vi "Set He Line Interlock Configuration.vi"(8 "error in (no error)":errorcluster, 9 "Manual Mode (False)":bool, 10 "Open? (False)":bool, 11 "He Line in":refnum<class "He Line.lvclass">) -> (0 "error out":errorcluster, 1 "Interlock Chain":refnum<class "Interlock Chain.lvclass">, 2 "Open? (False) 2":bool, 3 "He Line out":refnum<class "He Line.lvclass">)   [LabVIEW 2015, in "cRIO-Carbondioxide.lvlib" / "CO2-Actor.lvlib" / "He Line.lvclass"]
uses:
  He Line.lvclass
  Interlocks/Interlock Chain/Interlock Chain.lvclass
  cRIO-CO2/cRIO-CO2.lvclass
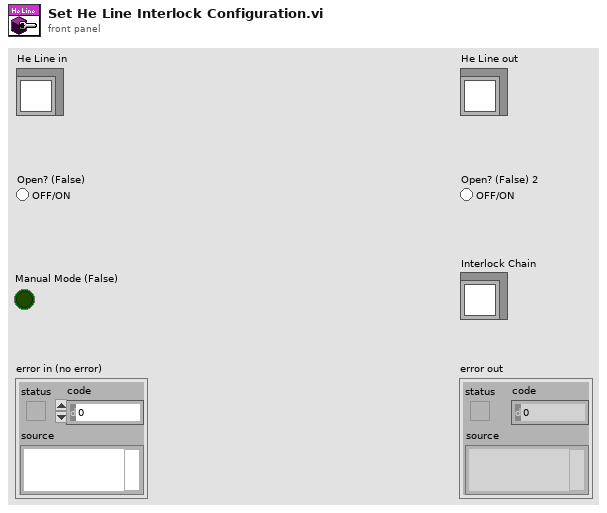
[diagram p1: front panel]
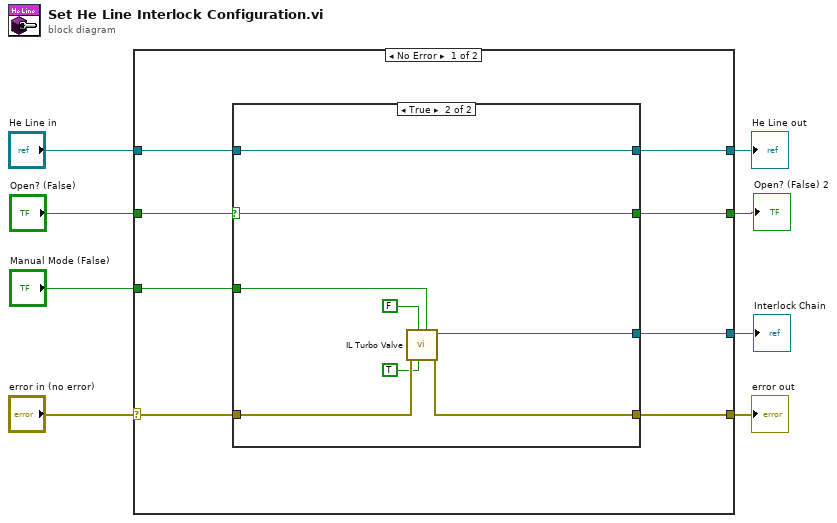
[diagram p0: block diagram]
diagram:
  n1 = case shown="No Error" "error in (no error)" {
    selector: "error in (no error)" -> [w16 w29]
    tunnel: [w15 w29] -> w7
    tunnel: [w11 w28] -> w5
    tunnel: "He Line in" -> [w12 w28]
    tunnel: "Open? (False)" -> [w10 _]
    tunnel: [w14 _] -> w3
    tunnel: "Manual Mode (False)" -> [w13 _]
    tunnel: [w9 _] -> w1
    frame No Error {
      n2 = case shown="True" w10 {
        selector: w10 -> [w17 w21]
        tunnel: w16 -> [w19 w27]
        tunnel: [w19 w26] -> w15
        tunnel: [_ w25] -> w14
        tunnel: w13 -> [_ w23]
        tunnel: w12 -> [w18 w22]
        tunnel: [w18 w22] -> w11
        tunnel: [w17 w21] -> w9
        frame False {
          # "Close Line. No Interlock"
        }
        frame True {
          n3 = call "IL Turbo Valve.vi"("Ignore (F)"=w23, "Interlock Condition (ON/OFF)"=TRUE, "Stop Self on IL? (T)"=FALSE, "error in (no error)"=w27) -> ("error out"=w26:errorcluster, "Interlock Chain out"=w25:refnum<class "Interlock Chain.lvclass">)  [unwired: 5 in, 1 out]
        }
      }
    }
    frame Error {
    }
  }
  "error out" <- w7
  "He Line out" <- w5
  "Interlock Chain" <- w3
  "Open? (False) 2" <- w1
